vi "resetAllChannels.vi"(8 "error in (no error)":errorcluster, 11 "AtomChipHWC in":refnum<class "AtomChipHWC.lvclass">) -> (0 "error out":errorcluster, 3 "AtomChipHWC out":refnum<class "AtomChipHWC.lvclass">)   [LabVIEW 2011, in "Hardware.lvlib" / "HWControllers.lvlib" / "AtomChipHWC.lvclass"]
uses:
  AtomChipHWC.lvclass
  AtomChipHWC.lvclass/AtomChipHWC.ctl
  Channels/VoltOutput/AnalogOutput.lvclass
  Channels/Digital/DigitalOutput.lvclass
  Channels/DDSOutput/Generic/DDSOutput.lvclass
  HWController.lvclass
  Tools/DatabaseHelpers/DbConnection/DeviceDataBase/deviceDataBase.lvclass
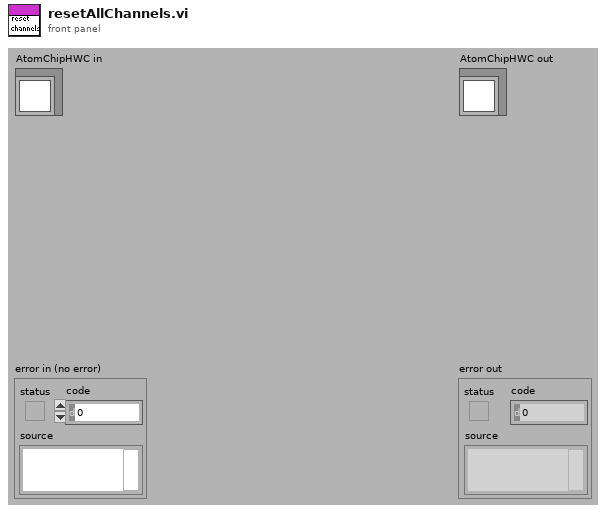
[diagram p1: front panel]
types:
  T1 = cluster{"VoltageLimit":dbl, "CurrentLimit":dbl}[]
  T2 = cluster{"Frequency(MHz)":dbl, "Amplitude":dbl, "Phase":dbl, "OutputForm":enum16{"Sine", "Square", "Triangle", "Arbitrary"}}[]
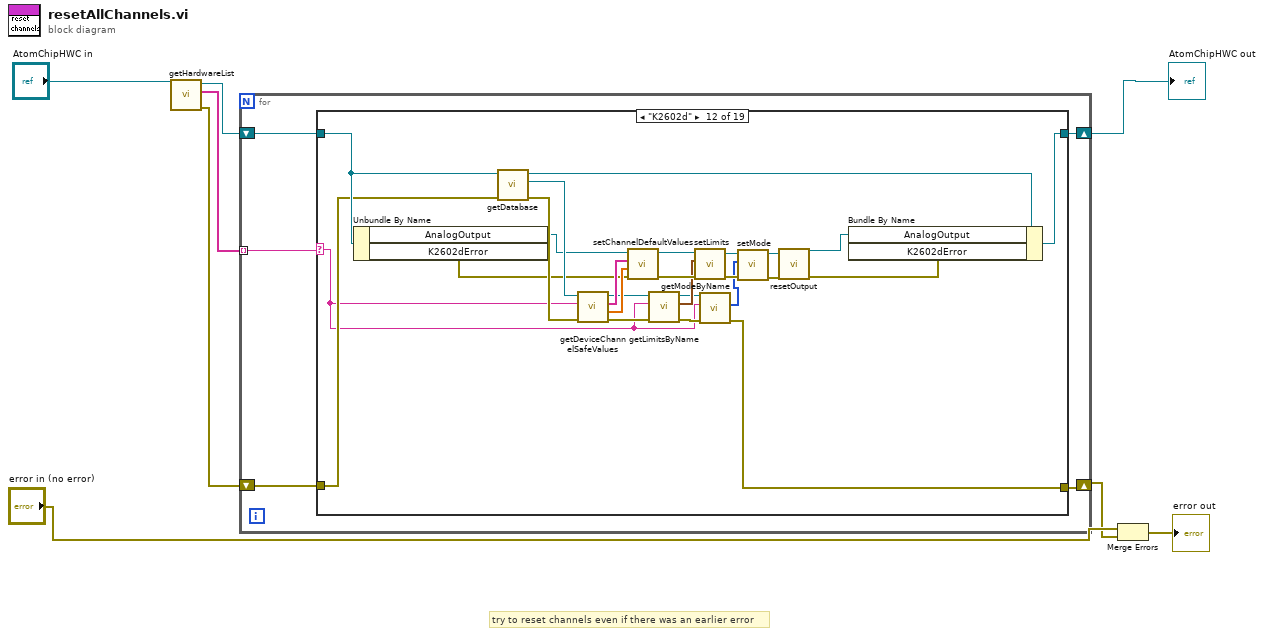
[diagram p0: block diagram]
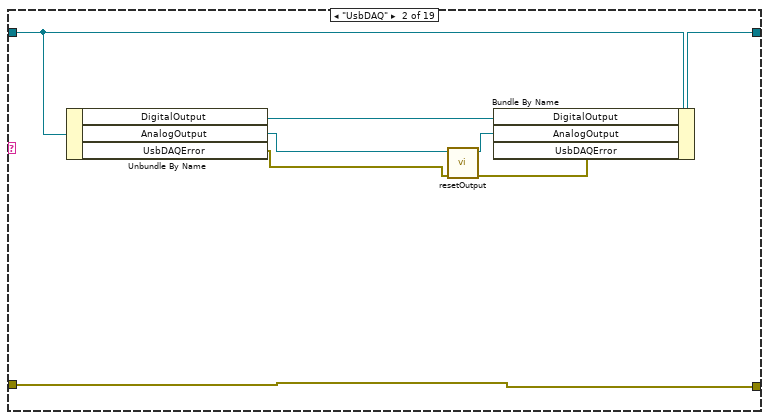
[diagram p3: hidden frame]
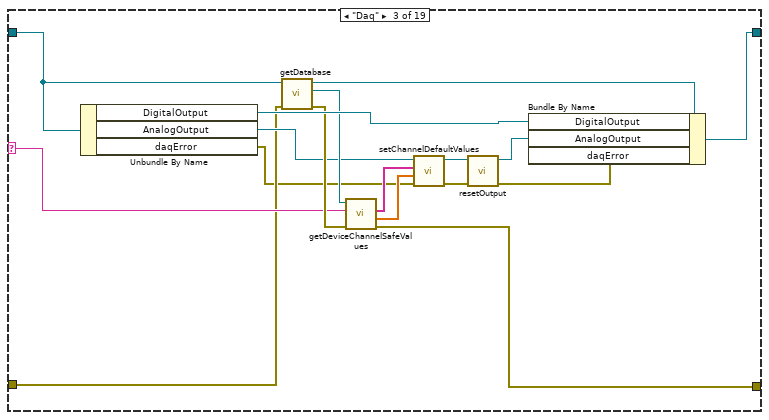
[diagram p4: hidden frame]
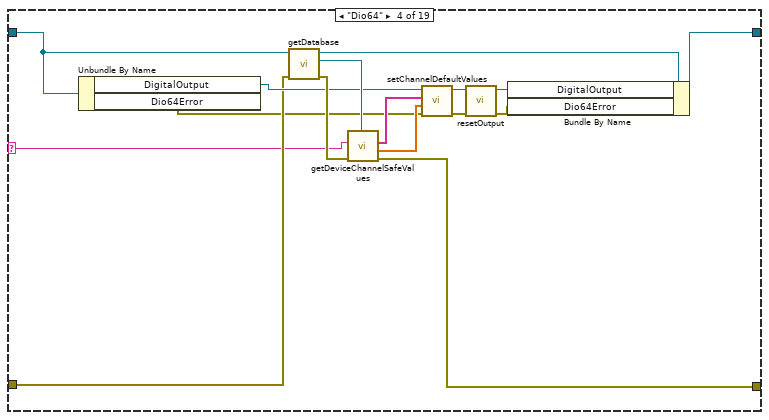
[diagram p5: hidden frame]
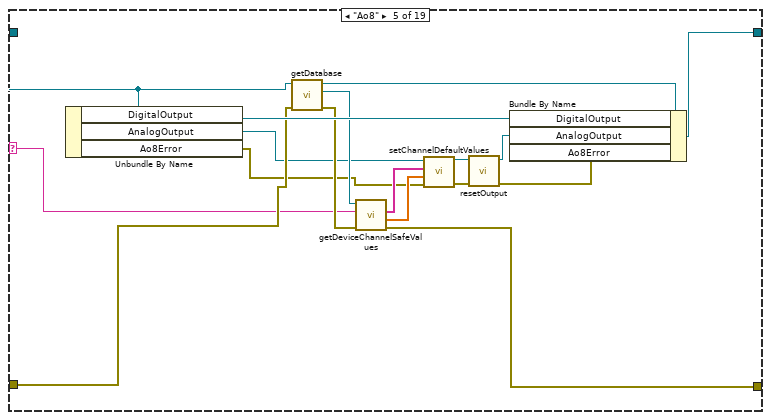
[diagram p6: hidden frame]
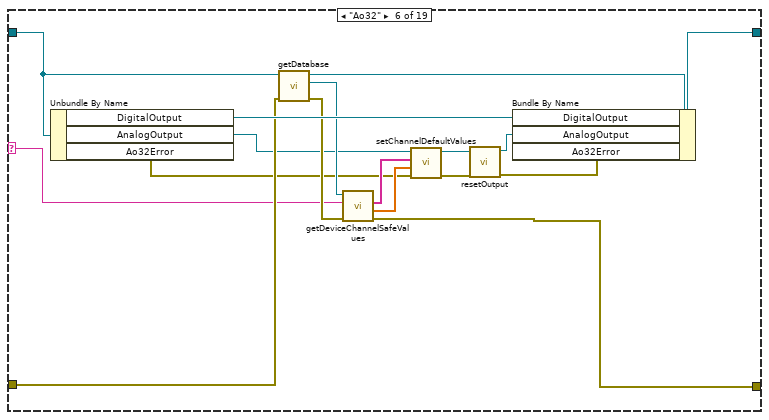
[diagram p7: hidden frame]
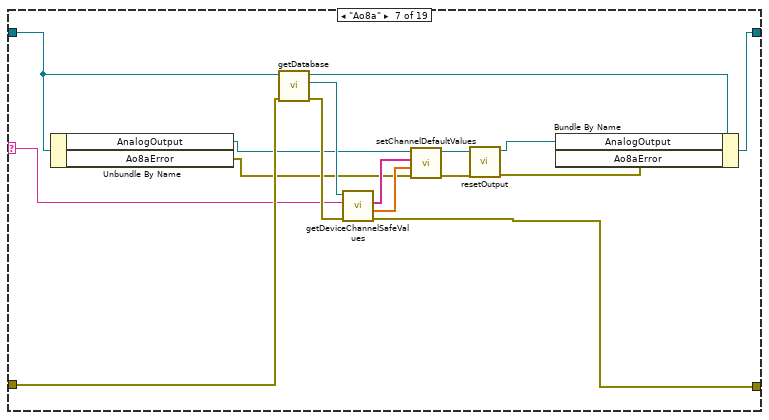
[diagram p8: hidden frame]
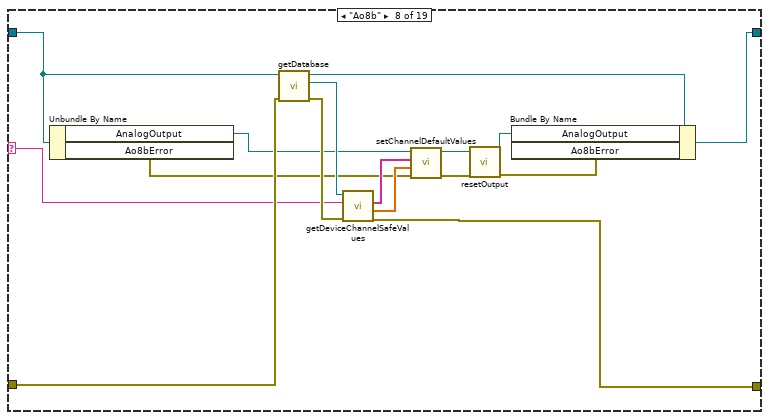
[diagram p9: hidden frame]
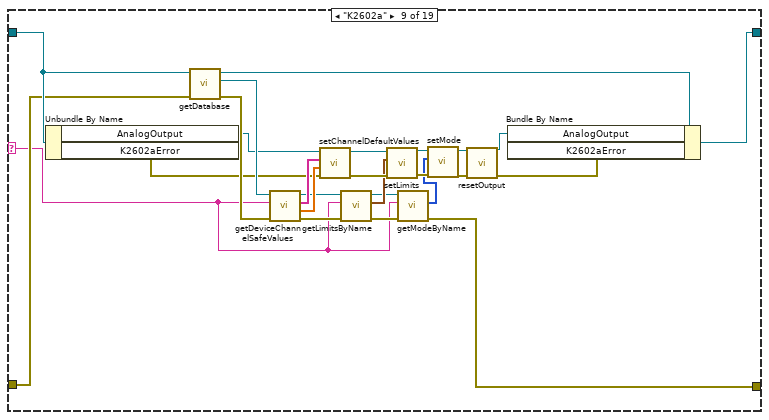
[diagram p10: hidden frame]
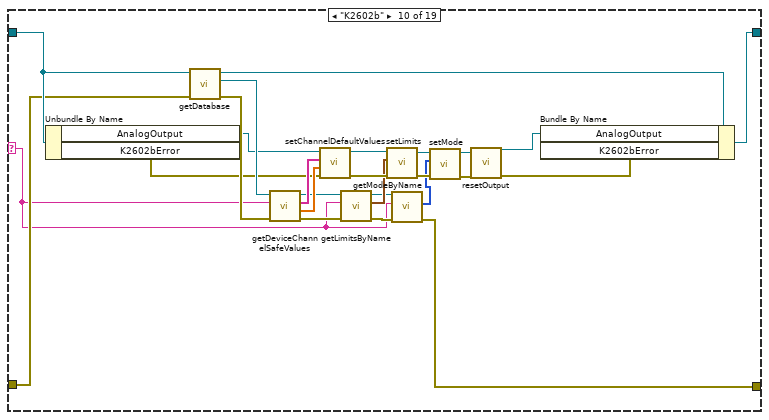
[diagram p11: hidden frame]
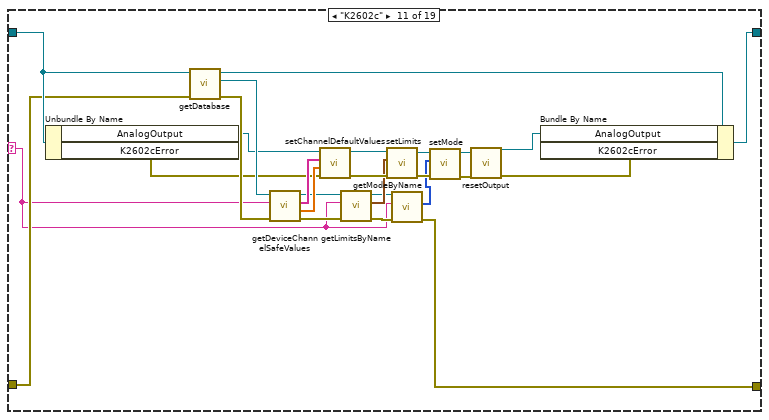
[diagram p12: hidden frame]
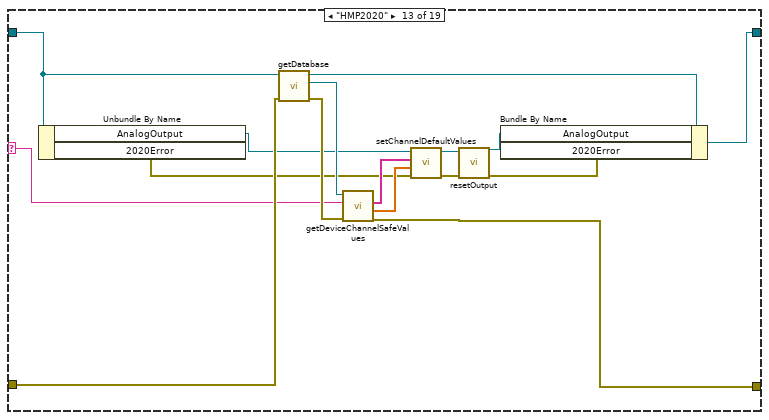
[diagram p13: hidden frame]
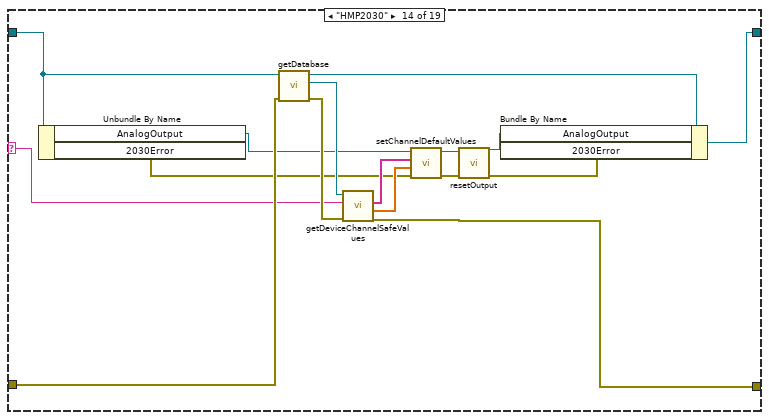
[diagram p14: hidden frame]
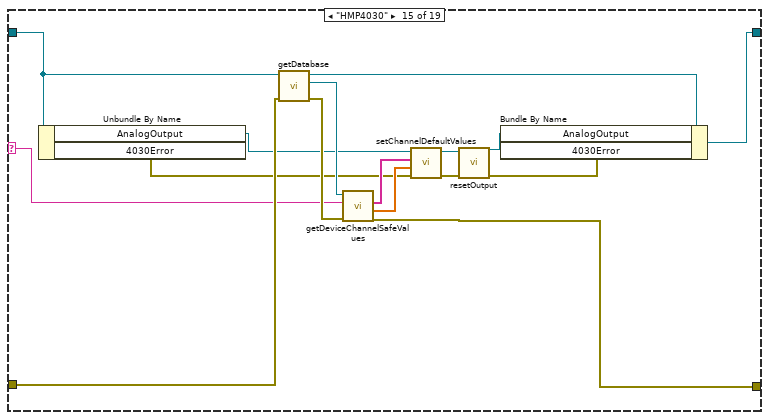
[diagram p15: hidden frame]
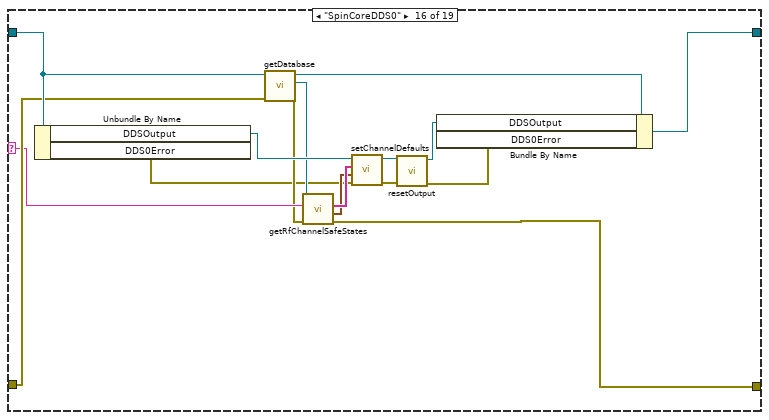
[diagram p16: hidden frame]
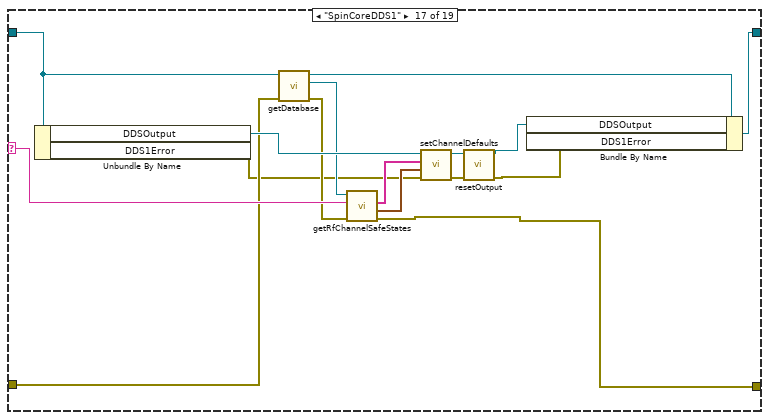
[diagram p17: hidden frame]
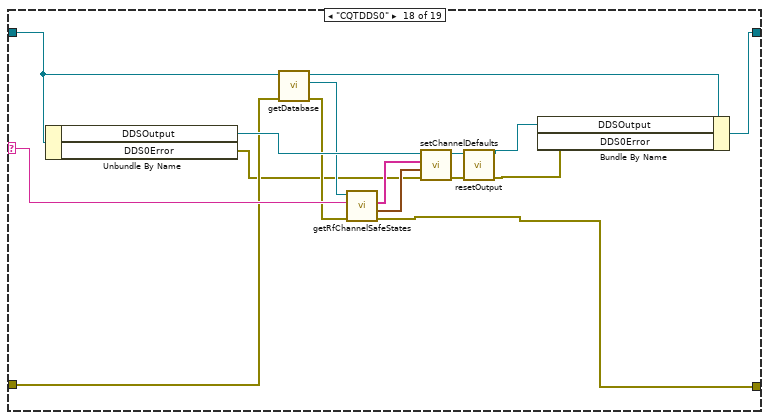
[diagram p18: hidden frame]
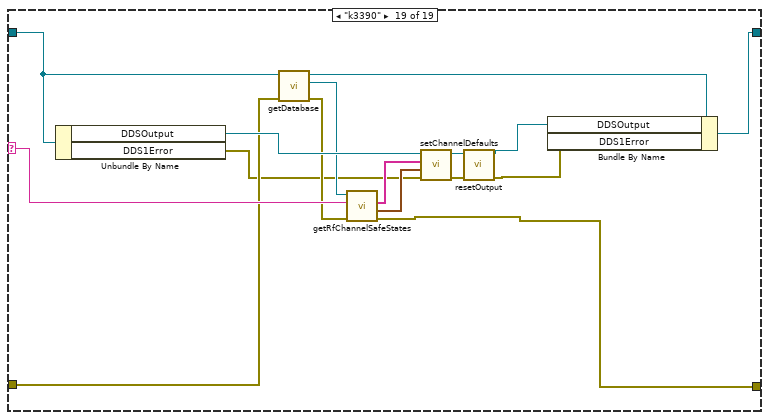
[diagram p19: hidden frame]
diagram:
  # "try to reset channels even if there was an earlier error"
  n1 = call "getHardwareList.vi"("HWController.lvclass in"="AtomChipHWC in") -> ("error out"=w4:errorcluster, "HardwareList"=w6:string[], "HWController.lvclass out"=w5:refnum<class "AtomChipHWC.lvclass">)  [unwired: 8 in]
  n2 = for {
    tunnel: w6 -> [w10] mode=indexing
    shift-right: [w13] -> w7
    shift-left: w5 -> [w9]
    shift-right: [w11] -> w1
    shift-left: w4 -> [w12]
    n3 = case shown="\"K2602d\"" w10 {
      selector: w10 -> [_ _ w29 w46 w62 w77 w94 w110 w129 w150 w176 w202 w230 w246 w262 w281 w298 w314 w330]
      tunnel: w9 -> [w15 w23 w31 w50 w66 w83 w100 w116 w142 w168 w194 w220 w236 w252 w268 w289 w305 w321 w337]
      tunnel: [w15 w22 w40 w56 w73 w90 w106 w122 w148 w174 w200 w226 w242 w258 w274 w290 w306 w322 w338] -> w13
      tunnel: w12 -> [w14 w16 w27 w47 w64 w82 w99 w115 w141 w167 w193 w219 w235 w251 w267 w288 w294 w310 w326]
      tunnel: [w14 w16 w26 w41 w57 w75 w92 w108 w123 w151 w177 w203 w228 w244 w260 w276 w292 w308 w324] -> w11
      frame "No Hardware", Default {
      }
      frame "UsbDAQ" {
        n4 = Unbundle By Name(w23) -> ("DigitalOutput"=w19:refnum<class "DigitalOutput.lvclass">, "AnalogOutput"=w21:refnum<class "AnalogOutput.lvclass">, "UsbDAQError"=w18:errorcluster)
        n5 = call-dynamic "resetOutput.vi"("error in (no error)"=w18, "AnalogOutput in"=w21) -> ("error out"=w17:errorcluster, "AnalogOutput out"=w20:refnum<class "AnalogOutput.lvclass">)  [unwired: 8 in]
        n6 = Bundle By Name(cluster=w23, "DigitalOutput"=w19, "AnalogOutput"=w20, "UsbDAQError"=w17) -> (w22:refnum<class "AtomChipHWC.lvclass">)
      }
      frame "Daq" {
        n7 = Unbundle By Name(w31) -> ("DigitalOutput"=w38:refnum<class "DigitalOutput.lvclass">, "AnalogOutput"=w32:refnum<class "AnalogOutput.lvclass">, "daqError"=w24:errorcluster)
        n8 = call "getDatabase.vi"("error in (no error)"=w27, "HWController in"=w31) -> ("error out"=w36:errorcluster, "deviceDataBase"=w37:refnum<class "deviceDataBase.lvclass">, "HWController out"=w30:refnum<class "AtomChipHWC.lvclass">)  [unwired: 7 in]
        n9 = call "getDeviceChannelSafeValues.vi"("error in (no error)"=w36, "device_name"=w29, "deviceDataBase in"=w37) -> ("error out"=w26:errorcluster, "SafeVaues"=w35:dbl[], "ChannelAddresses"=w34:string[])  [unwired: 5 in, 1 out]
        n10 = call "setChannelDefaultValues.vi"("error in (no error)"=w24, "calibratedValues"=w35, "channel_addresses"=w34, "AnalogOutput in"=w32) -> ("error out"=w28:errorcluster, "AnalogOutput out"=w33:refnum<class "AnalogOutput.lvclass">)  [unwired: 6 in]
        n11 = call-dynamic "resetOutput.vi"("error in (no error)"=w28, "AnalogOutput in"=w33) -> ("error out"=w25:errorcluster, "AnalogOutput out"=w39:refnum<class "AnalogOutput.lvclass">)  [unwired: 8 in]
        n12 = Bundle By Name(cluster=w30, "DigitalOutput"=w38, "AnalogOutput"=w39, "daqError"=w25) -> (w40:refnum<class "AtomChipHWC.lvclass">)
      }
      frame "Dio64" {
        n13 = Unbundle By Name(w50) -> ("DigitalOutput"=w48:refnum<class "DigitalOutput.lvclass">, "Dio64Error"=w43:errorcluster)
        n14 = call "getDatabase.vi"("error in (no error)"=w47, "HWController in"=w50) -> ("error out"=w53:errorcluster, "deviceDataBase"=w54:refnum<class "deviceDataBase.lvclass">, "HWController out"=w49:refnum<class "AtomChipHWC.lvclass">)  [unwired: 7 in]
        n15 = call "getDeviceChannelSafeValues.vi"("error in (no error)"=w53, "device_name"=w46, "deviceDataBase in"=w54) -> ("error out"=w41:errorcluster, "SafeVaues"=w51:dbl[], "ChannelAddresses"=w52:string[])  [unwired: 5 in, 1 out]
        n16 = call-dynamic "setChannelDefaultValues.vi"("error in (no error)"=w43, "calibratedValues"=w51, "channel_addresses"=w52, "DigitalOutput in"=w48) -> ("error out"=w45:errorcluster, "DigitalOutput out"=w44:refnum<class "DigitalOutput.lvclass">)  [unwired: 6 in]
        n17 = call-dynamic "resetOutput.vi"("error in (no error)"=w45, "DigitalOutput in"=w44) -> ("error out"=w42:errorcluster, "DigitalOutput out"=w55:refnum<class "DigitalOutput.lvclass">)  [unwired: 8 in]
        n18 = Bundle By Name(cluster=w49, "DigitalOutput"=w55, "Dio64Error"=w42) -> (w56:refnum<class "AtomChipHWC.lvclass">)
      }
      frame "Ao8" {
        n19 = Unbundle By Name(w66) -> ("DigitalOutput"=w71:refnum<class "DigitalOutput.lvclass">, "AnalogOutput"=w63:refnum<class "AnalogOutput.lvclass">, "Ao8Error"=w58:errorcluster)
        n20 = call "getDatabase.vi"("error in (no error)"=w64, "HWController in"=w66) -> ("error out"=w69:errorcluster, "deviceDataBase"=w70:refnum<class "deviceDataBase.lvclass">, "HWController out"=w65:refnum<class "AtomChipHWC.lvclass">)  [unwired: 7 in]
        n21 = call "getDeviceChannelSafeValues.vi"("error in (no error)"=w69, "device_name"=w62, "deviceDataBase in"=w70) -> ("error out"=w57:errorcluster, "SafeVaues"=w68:dbl[], "ChannelAddresses"=w67:string[])  [unwired: 5 in, 1 out]
        n22 = call "setChannelDefaultValues.vi"("error in (no error)"=w58, "calibratedValues"=w68, "channel_addresses"=w67, "AnalogOutput in"=w63) -> ("error out"=w60:errorcluster, "AnalogOutput out"=w61:refnum<class "AnalogOutput.lvclass">)  [unwired: 6 in]
        n23 = call-dynamic "resetOutput.vi"("error in (no error)"=w60, "AnalogOutput in"=w61) -> ("error out"=w59:errorcluster, "AnalogOutput out"=w72:refnum<class "AnalogOutput.lvclass">)  [unwired: 8 in]
        n24 = Bundle By Name(cluster=w65, "DigitalOutput"=w71, "AnalogOutput"=w72, "Ao8Error"=w59) -> (w73:refnum<class "AtomChipHWC.lvclass">)
      }
      frame "Ao32" {
        n25 = Unbundle By Name(w83) -> ("DigitalOutput"=w88:refnum<class "DigitalOutput.lvclass">, "AnalogOutput"=w80:refnum<class "AnalogOutput.lvclass">, "Ao32Error"=w76:errorcluster)
        n26 = call "getDatabase.vi"("error in (no error)"=w82, "HWController in"=w83) -> ("error out"=w86:errorcluster, "deviceDataBase"=w87:refnum<class "deviceDataBase.lvclass">, "HWController out"=w79:refnum<class "AtomChipHWC.lvclass">)  [unwired: 7 in]
        n27 = call "getDeviceChannelSafeValues.vi"("error in (no error)"=w86, "device_name"=w77, "deviceDataBase in"=w87) -> ("error out"=w75:errorcluster, "SafeVaues"=w85:dbl[], "ChannelAddresses"=w84:string[])  [unwired: 5 in, 1 out]
        n28 = call "setChannelDefaultValues.vi"("error in (no error)"=w76, "calibratedValues"=w85, "channel_addresses"=w84, "AnalogOutput in"=w80) -> ("error out"=w81:errorcluster, "AnalogOutput out"=w78:refnum<class "AnalogOutput.lvclass">)  [unwired: 6 in]
        n29 = call-dynamic "resetOutput.vi"("error in (no error)"=w81, "AnalogOutput in"=w78) -> ("error out"=w74:errorcluster, "AnalogOutput out"=w89:refnum<class "AnalogOutput.lvclass">)  [unwired: 8 in]
        n30 = Bundle By Name(cluster=w79, "DigitalOutput"=w88, "AnalogOutput"=w89, "Ao32Error"=w74) -> (w90:refnum<class "AtomChipHWC.lvclass">)
      }
      frame "Ao8a" {
        n31 = Unbundle By Name(w100) -> ("AnalogOutput"=w97:refnum<class "AnalogOutput.lvclass">, "Ao8aError"=w93:errorcluster)
        n32 = call "getDatabase.vi"("error in (no error)"=w99, "HWController in"=w100) -> ("error out"=w103:errorcluster, "deviceDataBase"=w104:refnum<class "deviceDataBase.lvclass">, "HWController out"=w96:refnum<class "AtomChipHWC.lvclass">)  [unwired: 7 in]
        n33 = call "getDeviceChannelSafeValues.vi"("error in (no error)"=w103, "device_name"=w94, "deviceDataBase in"=w104) -> ("error out"=w92:errorcluster, "SafeVaues"=w102:dbl[], "ChannelAddresses"=w101:string[])  [unwired: 5 in, 1 out]
        n34 = call "setChannelDefaultValues.vi"("error in (no error)"=w93, "calibratedValues"=w102, "channel_addresses"=w101, "AnalogOutput in"=w97) -> ("error out"=w98:errorcluster, "AnalogOutput out"=w95:refnum<class "AnalogOutput.lvclass">)  [unwired: 6 in]
        n35 = call-dynamic "resetOutput.vi"("error in (no error)"=w98, "AnalogOutput in"=w95) -> ("error out"=w91:errorcluster, "AnalogOutput out"=w105:refnum<class "AnalogOutput.lvclass">)  [unwired: 8 in]
        n36 = Bundle By Name(cluster=w96, "AnalogOutput"=w105, "Ao8aError"=w91) -> (w106:refnum<class "AtomChipHWC.lvclass">)
      }
      frame "Ao8b" {
        n37 = Unbundle By Name(w116) -> ("AnalogOutput"=w113:refnum<class "AnalogOutput.lvclass">, "Ao8bError"=w109:errorcluster)
        n38 = call "getDatabase.vi"("error in (no error)"=w115, "HWController in"=w116) -> ("error out"=w119:errorcluster, "deviceDataBase"=w120:refnum<class "deviceDataBase.lvclass">, "HWController out"=w112:refnum<class "AtomChipHWC.lvclass">)  [unwired: 7 in]
        n39 = call "getDeviceChannelSafeValues.vi"("error in (no error)"=w119, "device_name"=w110, "deviceDataBase in"=w120) -> ("error out"=w108:errorcluster, "SafeVaues"=w118:dbl[], "ChannelAddresses"=w117:string[])  [unwired: 5 in, 1 out]
        n40 = call "setChannelDefaultValues.vi"("error in (no error)"=w109, "calibratedValues"=w118, "channel_addresses"=w117, "AnalogOutput in"=w113) -> ("error out"=w114:errorcluster, "AnalogOutput out"=w111:refnum<class "AnalogOutput.lvclass">)  [unwired: 6 in]
        n41 = call-dynamic "resetOutput.vi"("error in (no error)"=w114, "AnalogOutput in"=w111) -> ("error out"=w107:errorcluster, "AnalogOutput out"=w121:refnum<class "AnalogOutput.lvclass">)  [unwired: 8 in]
        n42 = Bundle By Name(cluster=w112, "AnalogOutput"=w121, "Ao8bError"=w107) -> (w122:refnum<class "AtomChipHWC.lvclass">)
      }
      frame "K2602a" {
        n43 = Unbundle By Name(w142) -> ("AnalogOutput"=w140:refnum<class "AnalogOutput.lvclass">, "K2602aError"=w138:errorcluster)
        n44 = call "getDatabase.vi"("error in (no error)"=w141, "HWController in"=w142) -> ("error out"=w145:errorcluster, "deviceDataBase"=w146:refnum<class "deviceDataBase.lvclass">, "HWController out"=w139:refnum<class "AtomChipHWC.lvclass">)  [unwired: 7 in]
        n45 = call "getDeviceChannelSafeValues.vi"("error in (no error)"=w145, "device_name"=w129, "deviceDataBase in"=w146) -> ("error out"=w136:errorcluster, "SafeVaues"=w144:dbl[], "ChannelAddresses"=w143:string[], "deviceDataBase out"=w135:refnum<class "deviceDataBase.lvclass">)  [unwired: 5 in]
        n46 = call "setChannelDefaultValues.vi"("error in (no error)"=w138, "calibratedValues"=w144, "channel_addresses"=w143, "AnalogOutput in"=w140) -> ("error out"=w133:errorcluster, "AnalogOutput out"=w134:refnum<class "AnalogOutput.lvclass">)  [unwired: 6 in]
        n47 = call "getLimitsByName.vi"("error in (no error)"=w136, "device_name"=w129, "deviceDataBase in"=w135) -> ("error out"=w130:errorcluster, "Limits"=w132:T1, "deviceDataBase out"=w131:refnum<class "deviceDataBase.lvclass">)  [unwired: 6 in]
        n48 = call "setLimits.vi"("error in (no error)"=w133, "Limits"=w132, "AnalogOutput in"=w134) -> ("error out"=w125:errorcluster, "AnalogOutput out"=w128:refnum<class "AnalogOutput.lvclass">)  [unwired: 7 in]
        n49 = call "getModeByName.vi"("error in (no error)"=w130, "device_name"=w129, "deviceDataBase in"=w131) -> ("error out"=w123:errorcluster, "mode"=w124:enum16{"current", "voltage"}[])  [unwired: 6 in, 1 out]
        n50 = call "setMode.vi"("error in (no error)"=w125, "mode"=w124, "AnalogOutput in"=w128) -> ("error out"=w126:errorcluster, "AnalogOutput out"=w127:refnum<class "AnalogOutput.lvclass">)  [unwired: 7 in]
        n51 = call-dynamic "resetOutput.vi"("error in (no error)"=w126, "AnalogOutput in"=w127) -> ("error out"=w137:errorcluster, "AnalogOutput out"=w147:refnum<class "AnalogOutput.lvclass">)  [unwired: 8 in]
        n52 = Bundle By Name(cluster=w139, "AnalogOutput"=w147, "K2602aError"=w137) -> (w148:refnum<class "AtomChipHWC.lvclass">)
      }
      frame "K2602b" {
        n53 = Unbundle By Name(w168) -> ("AnalogOutput"=w166:refnum<class "AnalogOutput.lvclass">, "K2602bError"=w164:errorcluster)
        n54 = call "getDatabase.vi"("error in (no error)"=w167, "HWController in"=w168) -> ("error out"=w171:errorcluster, "deviceDataBase"=w172:refnum<class "deviceDataBase.lvclass">, "HWController out"=w165:refnum<class "AtomChipHWC.lvclass">)  [unwired: 7 in]
        n55 = call "getDeviceChannelSafeValues.vi"("error in (no error)"=w171, "device_name"=w150, "deviceDataBase in"=w172) -> ("error out"=w162:errorcluster, "SafeVaues"=w170:dbl[], "ChannelAddresses"=w169:string[], "deviceDataBase out"=w161:refnum<class "deviceDataBase.lvclass">)  [unwired: 5 in]
        n56 = call "setChannelDefaultValues.vi"("error in (no error)"=w164, "calibratedValues"=w170, "channel_addresses"=w169, "AnalogOutput in"=w166) -> ("error out"=w159:errorcluster, "AnalogOutput out"=w160:refnum<class "AnalogOutput.lvclass">)  [unwired: 6 in]
        n57 = call "getLimitsByName.vi"("error in (no error)"=w162, "device_name"=w150, "deviceDataBase in"=w161) -> ("error out"=w152:errorcluster, "Limits"=w158:T1, "deviceDataBase out"=w153:refnum<class "deviceDataBase.lvclass">)  [unwired: 6 in]
        n58 = call "setLimits.vi"("error in (no error)"=w159, "Limits"=w158, "AnalogOutput in"=w160) -> ("error out"=w156:errorcluster, "AnalogOutput out"=w157:refnum<class "AnalogOutput.lvclass">)  [unwired: 7 in]
        n59 = call "getModeByName.vi"("error in (no error)"=w152, "device_name"=w150, "deviceDataBase in"=w153) -> ("error out"=w151:errorcluster, "mode"=w149:enum16{"current", "voltage"}[])  [unwired: 6 in, 1 out]
        n60 = call "setMode.vi"("error in (no error)"=w156, "mode"=w149, "AnalogOutput in"=w157) -> ("error out"=w155:errorcluster, "AnalogOutput out"=w154:refnum<class "AnalogOutput.lvclass">)  [unwired: 7 in]
        n61 = call-dynamic "resetOutput.vi"("error in (no error)"=w155, "AnalogOutput in"=w154) -> ("error out"=w163:errorcluster, "AnalogOutput out"=w173:refnum<class "AnalogOutput.lvclass">)  [unwired: 8 in]
        n62 = Bundle By Name(cluster=w165, "AnalogOutput"=w173, "K2602bError"=w163) -> (w174:refnum<class "AtomChipHWC.lvclass">)
      }
      frame "K2602c" {
        n63 = Unbundle By Name(w194) -> ("AnalogOutput"=w192:refnum<class "AnalogOutput.lvclass">, "K2602cError"=w190:errorcluster)
        n64 = call "getDatabase.vi"("error in (no error)"=w193, "HWController in"=w194) -> ("error out"=w197:errorcluster, "deviceDataBase"=w198:refnum<class "deviceDataBase.lvclass">, "HWController out"=w191:refnum<class "AtomChipHWC.lvclass">)  [unwired: 7 in]
        n65 = call "getDeviceChannelSafeValues.vi"("error in (no error)"=w197, "device_name"=w176, "deviceDataBase in"=w198) -> ("error out"=w188:errorcluster, "SafeVaues"=w196:dbl[], "ChannelAddresses"=w195:string[], "deviceDataBase out"=w187:refnum<class "deviceDataBase.lvclass">)  [unwired: 5 in]
        n66 = call "setChannelDefaultValues.vi"("error in (no error)"=w190, "calibratedValues"=w196, "channel_addresses"=w195, "AnalogOutput in"=w192) -> ("error out"=w185:errorcluster, "AnalogOutput out"=w186:refnum<class "AnalogOutput.lvclass">)  [unwired: 6 in]
        n67 = call "getLimitsByName.vi"("error in (no error)"=w188, "device_name"=w176, "deviceDataBase in"=w187) -> ("error out"=w178:errorcluster, "Limits"=w184:T1, "deviceDataBase out"=w179:refnum<class "deviceDataBase.lvclass">)  [unwired: 6 in]
        n68 = call "setLimits.vi"("error in (no error)"=w185, "Limits"=w184, "AnalogOutput in"=w186) -> ("error out"=w182:errorcluster, "AnalogOutput out"=w183:refnum<class "AnalogOutput.lvclass">)  [unwired: 7 in]
        n69 = call "getModeByName.vi"("error in (no error)"=w178, "device_name"=w176, "deviceDataBase in"=w179) -> ("error out"=w177:errorcluster, "mode"=w175:enum16{"current", "voltage"}[])  [unwired: 6 in, 1 out]
        n70 = call "setMode.vi"("error in (no error)"=w182, "mode"=w175, "AnalogOutput in"=w183) -> ("error out"=w181:errorcluster, "AnalogOutput out"=w180:refnum<class "AnalogOutput.lvclass">)  [unwired: 7 in]
        n71 = call-dynamic "resetOutput.vi"("error in (no error)"=w181, "AnalogOutput in"=w180) -> ("error out"=w189:errorcluster, "AnalogOutput out"=w199:refnum<class "AnalogOutput.lvclass">)  [unwired: 8 in]
        n72 = Bundle By Name(cluster=w191, "AnalogOutput"=w199, "K2602cError"=w189) -> (w200:refnum<class "AtomChipHWC.lvclass">)
      }
      frame "K2602d" {
        n73 = Unbundle By Name(w220) -> ("AnalogOutput"=w218:refnum<class "AnalogOutput.lvclass">, "K2602dError"=w216:errorcluster)
        n74 = call "getDatabase.vi"("error in (no error)"=w219, "HWController in"=w220) -> ("error out"=w223:errorcluster, "deviceDataBase"=w224:refnum<class "deviceDataBase.lvclass">, "HWController out"=w217:refnum<class "AtomChipHWC.lvclass">)  [unwired: 7 in]
        n75 = call "getDeviceChannelSafeValues.vi"("error in (no error)"=w223, "device_name"=w202, "deviceDataBase in"=w224) -> ("error out"=w214:errorcluster, "SafeVaues"=w222:dbl[], "ChannelAddresses"=w221:string[], "deviceDataBase out"=w213:refnum<class "deviceDataBase.lvclass">)  [unwired: 5 in]
        n76 = call "setChannelDefaultValues.vi"("error in (no error)"=w216, "calibratedValues"=w222, "channel_addresses"=w221, "AnalogOutput in"=w218) -> ("error out"=w211:errorcluster, "AnalogOutput out"=w212:refnum<class "AnalogOutput.lvclass">)  [unwired: 6 in]
        n77 = call "getLimitsByName.vi"("error in (no error)"=w214, "device_name"=w202, "deviceDataBase in"=w213) -> ("error out"=w204:errorcluster, "Limits"=w210:T1, "deviceDataBase out"=w205:refnum<class "deviceDataBase.lvclass">)  [unwired: 6 in]
        n78 = call "setLimits.vi"("error in (no error)"=w211, "Limits"=w210, "AnalogOutput in"=w212) -> ("error out"=w208:errorcluster, "AnalogOutput out"=w209:refnum<class "AnalogOutput.lvclass">)  [unwired: 7 in]
        n79 = call "getModeByName.vi"("error in (no error)"=w204, "device_name"=w202, "deviceDataBase in"=w205) -> ("error out"=w203:errorcluster, "mode"=w201:enum16{"current", "voltage"}[])  [unwired: 6 in, 1 out]
        n80 = call "setMode.vi"("error in (no error)"=w208, "mode"=w201, "AnalogOutput in"=w209) -> ("error out"=w207:errorcluster, "AnalogOutput out"=w206:refnum<class "AnalogOutput.lvclass">)  [unwired: 7 in]
        n81 = call-dynamic "resetOutput.vi"("error in (no error)"=w207, "AnalogOutput in"=w206) -> ("error out"=w215:errorcluster, "AnalogOutput out"=w225:refnum<class "AnalogOutput.lvclass">)  [unwired: 8 in]
        n82 = Bundle By Name(cluster=w217, "AnalogOutput"=w225, "K2602dError"=w215) -> (w226:refnum<class "AtomChipHWC.lvclass">)
      }
      frame "HMP2020" {
        n83 = Unbundle By Name(w236) -> ("AnalogOutput"=w233:refnum<class "AnalogOutput.lvclass">, "2020Error"=w229:errorcluster)
        n84 = call "getDatabase.vi"("error in (no error)"=w235, "HWController in"=w236) -> ("error out"=w239:errorcluster, "deviceDataBase"=w240:refnum<class "deviceDataBase.lvclass">, "HWController out"=w232:refnum<class "AtomChipHWC.lvclass">)  [unwired: 7 in]
        n85 = call "getDeviceChannelSafeValues.vi"("error in (no error)"=w239, "device_name"=w230, "deviceDataBase in"=w240) -> ("error out"=w228:errorcluster, "SafeVaues"=w238:dbl[], "ChannelAddresses"=w237:string[])  [unwired: 5 in, 1 out]
        n86 = call "setChannelDefaultValues.vi"("error in (no error)"=w229, "calibratedValues"=w238, "channel_addresses"=w237, "AnalogOutput in"=w233) -> ("error out"=w234:errorcluster, "AnalogOutput out"=w231:refnum<class "AnalogOutput.lvclass">)  [unwired: 6 in]
        n87 = call-dynamic "resetOutput.vi"("error in (no error)"=w234, "AnalogOutput in"=w231) -> ("error out"=w227:errorcluster, "AnalogOutput out"=w241:refnum<class "AnalogOutput.lvclass">)  [unwired: 8 in]
        n88 = Bundle By Name(cluster=w232, "AnalogOutput"=w241, "2020Error"=w227) -> (w242:refnum<class "AtomChipHWC.lvclass">)
      }
      frame "HMP2030" {
        n89 = Unbundle By Name(w252) -> ("AnalogOutput"=w249:refnum<class "AnalogOutput.lvclass">, "2030Error"=w245:errorcluster)
        n90 = call "getDatabase.vi"("error in (no error)"=w251, "HWController in"=w252) -> ("error out"=w255:errorcluster, "deviceDataBase"=w256:refnum<class "deviceDataBase.lvclass">, "HWController out"=w248:refnum<class "AtomChipHWC.lvclass">)  [unwired: 7 in]
        n91 = call "getDeviceChannelSafeValues.vi"("error in (no error)"=w255, "device_name"=w246, "deviceDataBase in"=w256) -> ("error out"=w244:errorcluster, "SafeVaues"=w254:dbl[], "ChannelAddresses"=w253:string[])  [unwired: 5 in, 1 out]
        n92 = call "setChannelDefaultValues.vi"("error in (no error)"=w245, "calibratedValues"=w254, "channel_addresses"=w253, "AnalogOutput in"=w249) -> ("error out"=w250:errorcluster, "AnalogOutput out"=w247:refnum<class "AnalogOutput.lvclass">)  [unwired: 6 in]
        n93 = call-dynamic "resetOutput.vi"("error in (no error)"=w250, "AnalogOutput in"=w247) -> ("error out"=w243:errorcluster, "AnalogOutput out"=w257:refnum<class "AnalogOutput.lvclass">)  [unwired: 8 in]
        n94 = Bundle By Name(cluster=w248, "AnalogOutput"=w257, "2030Error"=w243) -> (w258:refnum<class "AtomChipHWC.lvclass">)
      }
      frame "HMP4030" {
        n95 = Unbundle By Name(w268) -> ("AnalogOutput"=w265:refnum<class "AnalogOutput.lvclass">, "4030Error"=w261:errorcluster)
        n96 = call "getDatabase.vi"("error in (no error)"=w267, "HWController in"=w268) -> ("error out"=w271:errorcluster, "deviceDataBase"=w272:refnum<class "deviceDataBase.lvclass">, "HWController out"=w264:refnum<class "AtomChipHWC.lvclass">)  [unwired: 7 in]
        n97 = call "getDeviceChannelSafeValues.vi"("error in (no error)"=w271, "device_name"=w262, "deviceDataBase in"=w272) -> ("error out"=w260:errorcluster, "SafeVaues"=w270:dbl[], "ChannelAddresses"=w269:string[])  [unwired: 5 in, 1 out]
        n98 = call "setChannelDefaultValues.vi"("error in (no error)"=w261, "calibratedValues"=w270, "channel_addresses"=w269, "AnalogOutput in"=w265) -> ("error out"=w266:errorcluster, "AnalogOutput out"=w263:refnum<class "AnalogOutput.lvclass">)  [unwired: 6 in]
        n99 = call-dynamic "resetOutput.vi"("error in (no error)"=w266, "AnalogOutput in"=w263) -> ("error out"=w259:errorcluster, "AnalogOutput out"=w273:refnum<class "AnalogOutput.lvclass">)  [unwired: 8 in]
        n100 = Bundle By Name(cluster=w264, "AnalogOutput"=w273, "4030Error"=w259) -> (w274:refnum<class "AtomChipHWC.lvclass">)
      }
      frame "SpinCoreDDS0" {
        n101 = Unbundle By Name(w289) -> ("DDSOutput"=w286:refnum<class "DDSOutput.lvclass">, "DDS0Error"=w277:errorcluster)
        n102 = call "getDatabase.vi"("error in (no error)"=w288, "HWController in"=w289) -> ("error out"=w280:errorcluster, "deviceDataBase"=w282:refnum<class "deviceDataBase.lvclass">, "HWController out"=w287:refnum<class "AtomChipHWC.lvclass">)  [unwired: 7 in]
        n103 = call "getRfChannelSafeStates.vi"("error in (no error)"=w280, "deviceName"=w281, "deviceDataBase in"=w282) -> ("error out"=w276:errorcluster, "safestates"=w278:T2, "ChannelAddresses"=w279:string[])  [unwired: 5 in, 1 out]
        n104 = call-dynamic "setChannelDefaults.vi"("error in (no error)"=w277, "Data"=w278, "physicalChannels"=w279, "DDSOutput in"=w286) -> ("error out"=w284:errorcluster, "DDSOutput out"=w285:refnum<class "DDSOutput.lvclass">)  [unwired: 6 in]
        n105 = call-dynamic "resetOutput.vi"("error in (no error)"=w284, "DDSOutput in"=w285) -> ("error out"=w275:errorcluster, "DDSOutput out"=w283:refnum<class "DDSOutput.lvclass">)  [unwired: 8 in]
        n106 = Bundle By Name(cluster=w287, "DDSOutput"=w283, "DDS0Error"=w275) -> (w290:refnum<class "AtomChipHWC.lvclass">)
      }
      frame "SpinCoreDDS1" {
        n107 = Unbundle By Name(w305) -> ("DDSOutput"=w303:refnum<class "DDSOutput.lvclass">, "DDS1Error"=w291:errorcluster)
        n108 = call "getDatabase.vi"("error in (no error)"=w294, "HWController in"=w305) -> ("error out"=w297:errorcluster, "deviceDataBase"=w299:refnum<class "deviceDataBase.lvclass">, "HWController out"=w304:refnum<class "AtomChipHWC.lvclass">)  [unwired: 7 in]
        n109 = call "getRfChannelSafeStates.vi"("error in (no error)"=w297, "deviceName"=w298, "deviceDataBase in"=w299) -> ("error out"=w292:errorcluster, "safestates"=w296:T2, "ChannelAddresses"=w295:string[])  [unwired: 5 in, 1 out]
        n110 = call-dynamic "setChannelDefaults.vi"("error in (no error)"=w291, "Data"=w296, "physicalChannels"=w295, "DDSOutput in"=w303) -> ("error out"=w301:errorcluster, "DDSOutput out"=w302:refnum<class "DDSOutput.lvclass">)  [unwired: 6 in]
        n111 = call-dynamic "resetOutput.vi"("error in (no error)"=w301, "DDSOutput in"=w302) -> ("error out"=w293:errorcluster, "DDSOutput out"=w300:refnum<class "DDSOutput.lvclass">)  [unwired: 8 in]
        n112 = Bundle By Name(cluster=w304, "DDSOutput"=w300, "DDS1Error"=w293) -> (w306:refnum<class "AtomChipHWC.lvclass">)
      }
      frame "CQTDDS0" {
        n113 = Unbundle By Name(w321) -> ("DDSOutput"=w319:refnum<class "DDSOutput.lvclass">, "DDS0Error"=w307:errorcluster)
        n114 = call "getDatabase.vi"("error in (no error)"=w310, "HWController in"=w321) -> ("error out"=w313:errorcluster, "deviceDataBase"=w315:refnum<class "deviceDataBase.lvclass">, "HWController out"=w320:refnum<class "AtomChipHWC.lvclass">)  [unwired: 7 in]
        n115 = call "getRfChannelSafeStates.vi"("error in (no error)"=w313, "deviceName"=w314, "deviceDataBase in"=w315) -> ("error out"=w308:errorcluster, "safestates"=w312:T2, "ChannelAddresses"=w311:string[])  [unwired: 5 in, 1 out]
        n116 = call-dynamic "setChannelDefaults.vi"("error in (no error)"=w307, "Data"=w312, "physicalChannels"=w311, "DDSOutput in"=w319) -> ("error out"=w317:errorcluster, "DDSOutput out"=w318:refnum<class "DDSOutput.lvclass">)  [unwired: 6 in]
        n117 = call-dynamic "resetOutput.vi"("error in (no error)"=w317, "DDSOutput in"=w318) -> ("error out"=w309:errorcluster, "DDSOutput out"=w316:refnum<class "DDSOutput.lvclass">)  [unwired: 8 in]
        n118 = Bundle By Name(cluster=w320, "DDSOutput"=w316, "DDS0Error"=w309) -> (w322:refnum<class "AtomChipHWC.lvclass">)
      }
      frame "k3390" {
        n119 = Unbundle By Name(w337) -> ("DDSOutput"=w335:refnum<class "DDSOutput.lvclass">, "DDS1Error"=w323:errorcluster)
        n120 = call "getDatabase.vi"("error in (no error)"=w326, "HWController in"=w337) -> ("error out"=w329:errorcluster, "deviceDataBase"=w331:refnum<class "deviceDataBase.lvclass">, "HWController out"=w336:refnum<class "AtomChipHWC.lvclass">)  [unwired: 7 in]
        n121 = call "getRfChannelSafeStates.vi"("error in (no error)"=w329, "deviceName"=w330, "deviceDataBase in"=w331) -> ("error out"=w324:errorcluster, "safestates"=w328:T2, "ChannelAddresses"=w327:string[])  [unwired: 5 in, 1 out]
        n122 = call-dynamic "setChannelDefaults.vi"("error in (no error)"=w323, "Data"=w328, "physicalChannels"=w327, "DDSOutput in"=w335) -> ("error out"=w333:errorcluster, "DDSOutput out"=w334:refnum<class "DDSOutput.lvclass">)  [unwired: 6 in]
        n123 = call-dynamic "resetOutput.vi"("error in (no error)"=w333, "DDSOutput in"=w334) -> ("error out"=w325:errorcluster, "DDSOutput out"=w332:refnum<class "DDSOutput.lvclass">)  [unwired: 8 in]
        n124 = Bundle By Name(cluster=w336, "DDSOutput"=w332, "DDS1Error"=w325) -> (w338:refnum<class "AtomChipHWC.lvclass">)
      }
    }
  }
  "AtomChipHWC out" <- w7
  n125 = Merge Errors("error in (no error)", w1) -> (→"error out":errorcluster)
